vi "forward_prop.vi"(3 "Y":dbl[][](array[numeric]), 4 "X":dbl[][](array[numeric]), 5 "b":dbl, 6 "W":dbl[][](array[numeric])) -> (0 "db":dbl, 1 "dw":dbl[][](array[numeric]), 2 "cost":dbl)   [LabVIEW 2020]
uses:
  <vilib>/Analysis/baseanly.llb/Real A x B.vi
  <vilib>/Analysis/Matrix/Numeric/Conversions/Array To Matrix - RA2.vi
  <vilib>/Analysis/Matrix/Numeric/Conversions/Matrix To Array - RM.vi
  <vilib>/Analysis/NI_AALBase.lvlib
  <vilib>/Analysis/Matrix/NI_Matrix.lvlib
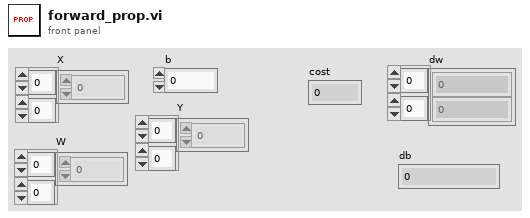
[diagram p1: front panel]
types:
  T1 = typedef "NI_Matrix.lvlib/RealMatrix.ctl" = dbl[][]
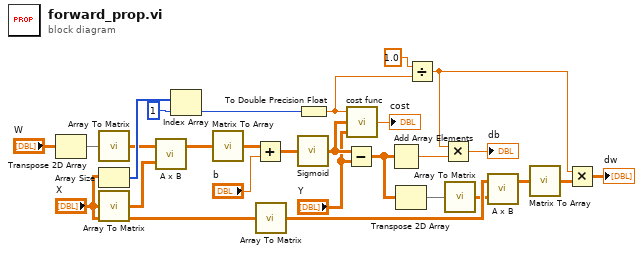
[diagram p0: block diagram]
diagram:
  n1 = Transpose 2D Array(2D array="W") -> (transposed array=w24:dbl[][])
  n2 = call-poly <vilib>:"Array To Matrix.vi"("Real 2D Array"=w24) -> ("Real Matrix"=w23:T1)
  n3 = Array Size(array="X") -> (size(s)=w27:i32[])
  n4 = call-poly <vilib>:"Array To Matrix.vi"("Real 2D Array"="X") -> ("Real Matrix"=w22:T1)
  n5 = call-poly <vilib>:"A x B.vi"("B"=w22, "A"=w23) -> ("A x B"=w21:T1)  [unwired: 1 out]
  n6 = Index Array(array=w27, index=1) -> (element=w16:i32)
  n7 = call-poly <vilib>:"Matrix To Array.vi"("Real Matrix"=w21) -> ("Real 2D Array"=w20:dbl[][])
  n8 = Add(x=w20, y="b") -> (x+y=w18:dbl[][])
  n9 = call-poly <vilib>:"Array To Matrix.vi"("Real 2D Array"="X") -> ("Real Matrix"=w9:T1)
  n10 = call "Sigmoid.vi"("Z"=w18) -> ("Sigmoid(Z)"=w13:dbl[][])  [unwired: 2 in]
  n11 = To Double Precision Float(number=w16) -> (double precision float=w15:dbl)
  n12 = Subtract(x=w13, y="Y") -> (x-y=w1:dbl[][])
  n13 = call "cost func.vi"("Y"="Y", "A"=w13, "m"=w15) -> ("cost"=→"cost":dbl)
  n14 = Add Array Elements(numeric array=w1) -> (sum=w11:dbl)
  n15 = Transpose 2D Array(2D array=w1) -> (transposed array=w2:dbl[][])
  n16 = Divide(x=1.0, y=w15) -> (x/y=w6:dbl)
  n17 = Multiply(x=w6, y=w11) -> (x*y=→"db":dbl)
  n18 = call-poly <vilib>:"Array To Matrix.vi"("Real 2D Array"=w2) -> ("Real Matrix"=w8:T1)
  n19 = call-poly <vilib>:"A x B.vi"("B"=w8, "A"=w9) -> ("A x B"=w7:T1)  [unwired: 1 out]
  n20 = call-poly <vilib>:"Matrix To Array.vi"("Real Matrix"=w7) -> ("Real 2D Array"=w5:dbl[][])
  n21 = Multiply(x=w6, y=w5) -> (x*y=→"dw":dbl[][])
